vi "Write Update Water Level Msg.vi"(10 "Update Water Level Msg":refnum<class "Update Water Level Msg.lvclass">, 11 "Water Level in":refnum<class "Water Level.lvclass">) -> (3 "Water Level out":refnum<class "Water Level.lvclass">)   [LabVIEW 2025, in "Water Level.lvlib" / "Water Level.lvclass"]
doc: "Writes the Update Water Level message that should be used to send updates about the water depth to the caller. Caller actors should set this *before* calling Launch Actor.vi."
uses:
  Water Level.lvclass
  Update Water Level Msg/Update Water Level Msg.lvclass
  Water Level.lvclass/Water Level.ctl
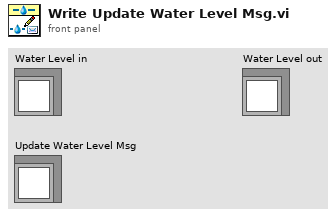
[diagram p1: front panel]
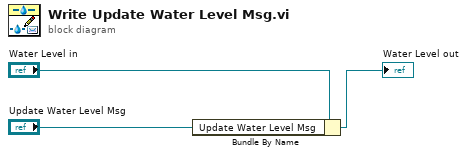
[diagram p0: block diagram]
diagram:
  n1 = Bundle By Name(cluster="Water Level in", "Update Water Level Msg"="Update Water Level Msg") -> (→"Water Level out":refnum<class "Water Level.lvclass">)
